vi "Example Button Callback.vi"() -> ()   [LabVIEW 2013]
uses:
  C:/tf/play/labview/Tinkerforge.dll
panel:
  out "last released":u8=255
  in  "stop":bool
  out "last pressed":u8=255
  in  "uid":string="SCD32"
  in  "port":i32=4223
  in  "host":string="localhost"
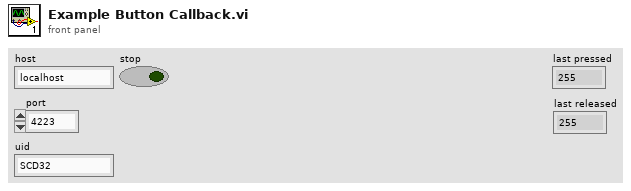
[diagram p1: front panel]
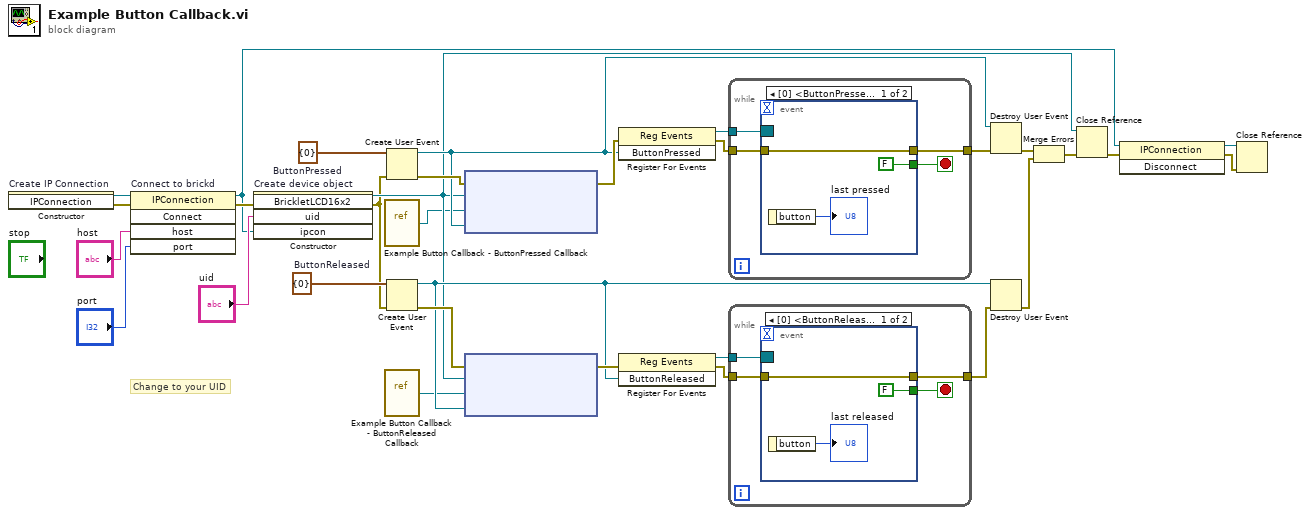
[diagram p0: block diagram]
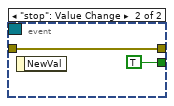
[diagram p2: hidden frame]
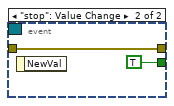
[diagram p3: hidden frame]
diagram:
  w5 = cluster{"button":u8} {"button"=0}  # ButtonReleased
  w16 = cluster{"button":u8} {"button"=0}  # ButtonPressed
  # "Change to your UID"
  n1 = constructor on="Create IP Connection" class="IPConnection"() -> (reference out=w31:refnum<k24>, error out=w1:errorcluster)  [unwired: 3 in, 1 out]
  n2 = invoke on="Connect to brickd" class="IPConnection" method="Connect"(reference=w31, error in=w1, "host"="host", "port"="port") -> (reference out=w24:refnum<k24>, error out=w27:errorcluster)  [unwired: 1 in, 3 out]
  n3 = constructor on="Create device object" class="BrickletLCD16x2"(error in=w27, "uid"="uid", "ipcon"=w24) -> (reference out=w6:refnum<k24>, error out=w4:errorcluster)  [unwired: 2 in, 3 out]
  n4 = vi-ref "Example Button Callback - ButtonPressed Callback.vi"() -> ("vi reference"=w3:refnum<vi>)
  n5 = vi-ref "Example Button Callback - ButtonReleased Callback.vi"() -> ("vi reference"=w2:refnum<vi>)
  n6 = Create User Event(user event datatype=w16, error in=w4) -> (user event=w17:refnum<user-event>, error out=w22:errorcluster)
  n7 = Create User Event(user event datatype=w5, error in=w4) -> (user event=w8:refnum<user-event>, error out=w13:errorcluster)
  n8 = node ("Register Event Callback")(w22, w6, w3, w17) -> (w21:errorcluster)  [unwired: 1 in, 1 out]
  n9 = node ("Register Event Callback")(w13, w6, w2, w8) -> (w12:errorcluster)  [unwired: 1 in, 1 out]
  n10 = register-events(error in=w21, w17) -> (reference out=w20:refnum<event-registration>, error out=w18:errorcluster)  [unwired: 1 in]
  n11 = register-events(error in=w12, w8) -> (reference out=w11:refnum<event-registration>, error out=w9:errorcluster)  [unwired: 1 in]
  n12 = while {
    tunnel: w20 -> [w35]
    tunnel: [w34] -> w19
    tunnel: w18 -> [w33]
    stop <- w32 stop-if-true
    n13 = event shown="[0] <ButtonPressed>: User Event" {
      selector: w35 -> [_ _]
      dyn-events: _ -> [_ _]
      timeout: _ -> [_ _]
      tunnel: [w38 w39] -> w34
      tunnel: w33 -> [w38 w39]
      tunnel: [FALSE TRUE] -> w32
      event User Event {
        n14 = event-data() -> ("button"=→"last pressed":u8)  [unwired: 1 in]
      }
      event "stop": Value Change {
        n15 = event-data() -> ()  [unwired: 1 in, 1 out]
      }
    }
  }
  n16 = while {
    tunnel: w11 -> [w44]
    tunnel: [w43] -> w10
    tunnel: w9 -> [w42]
    stop <- w41 stop-if-true
    n17 = event shown="[0] <ButtonReleased>: User Event" {
      selector: w44 -> [_ _]
      dyn-events: _ -> [_ _]
      timeout: _ -> [_ _]
      tunnel: [w47 w48] -> w43
      tunnel: w42 -> [w47 w48]
      tunnel: [FALSE TRUE] -> w41
      event User Event {
        n18 = event-data() -> ("button"=→"last released":u8)  [unwired: 1 in]
      }
      event "stop": Value Change {
        n19 = event-data() -> ()  [unwired: 1 in, 1 out]
      }
    }
  }
  n20 = Destroy User Event(user event=w17, error in=w19) -> (error out=w15:errorcluster)
  n21 = Destroy User Event(user event=w8, error in=w10) -> (error out=w7:errorcluster)
  n22 = Merge Errors(w15, w7) -> (w14:errorcluster)
  n23 = Close Reference(reference=w6, error in (no error)=w14) -> (error out=w26:errorcluster)
  n24 = invoke class="IPConnection" method="Disconnect"(reference=w24, error in=w26) -> (reference out=w23:refnum<k24>, error out=w25:errorcluster)  [unwired: 1 in, 1 out]
  n25 = Close Reference(reference=w23, error in (no error)=w25) -> ()  [unwired: 1 out]
